vi "Change.vi"(6 "OldVal":variant, 8 "error in (no error)":errorcluster, 9 "NewVal":variant, 10 "Control Index":i32=-1, 11 "UndoObject in":refnum<class "UndoObject.lvclass">) -> (0 "error out":errorcluster, 1 "Redo Enable":bool, 2 "Undo Enable":bool, 3 "UndoObject out":refnum<class "UndoObject.lvclass">)   [LabVIEW 2015, in "UndoLibrary.lvlib" / "UndoObject.lvclass"]
doc: "This VI stores the changes produced in the controls. The maximum number of change is corresponding to the size of the buffer."
uses:
  UndoObject.lvclass
  UndoObject.lvclass/UndoObject.ctl
  Support VIs/DataClass/Controls/cluster_Control Value.ctl
  Support VIs/DataClass/DataObject.lvclass/DataObject.ctl
  <vilib>/Utility/error.llb/Error Cluster From Error Code.vi
  <vilib>/ErrorRing/Error Ring.xnode
  Support VIs/DataClass/DataObject.lvclass
  QueueOperations/QueueOperations.lvlib
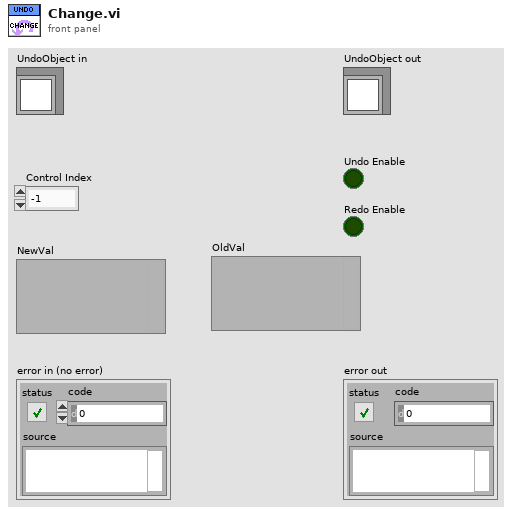
[diagram p1: front panel]
types:
  T1 = typedef "UndoLibrary.lvlib/DataObject.lvclass/cluster_Control Value.ctl" = cluster{"Index":i32, "Variant Data":variant}
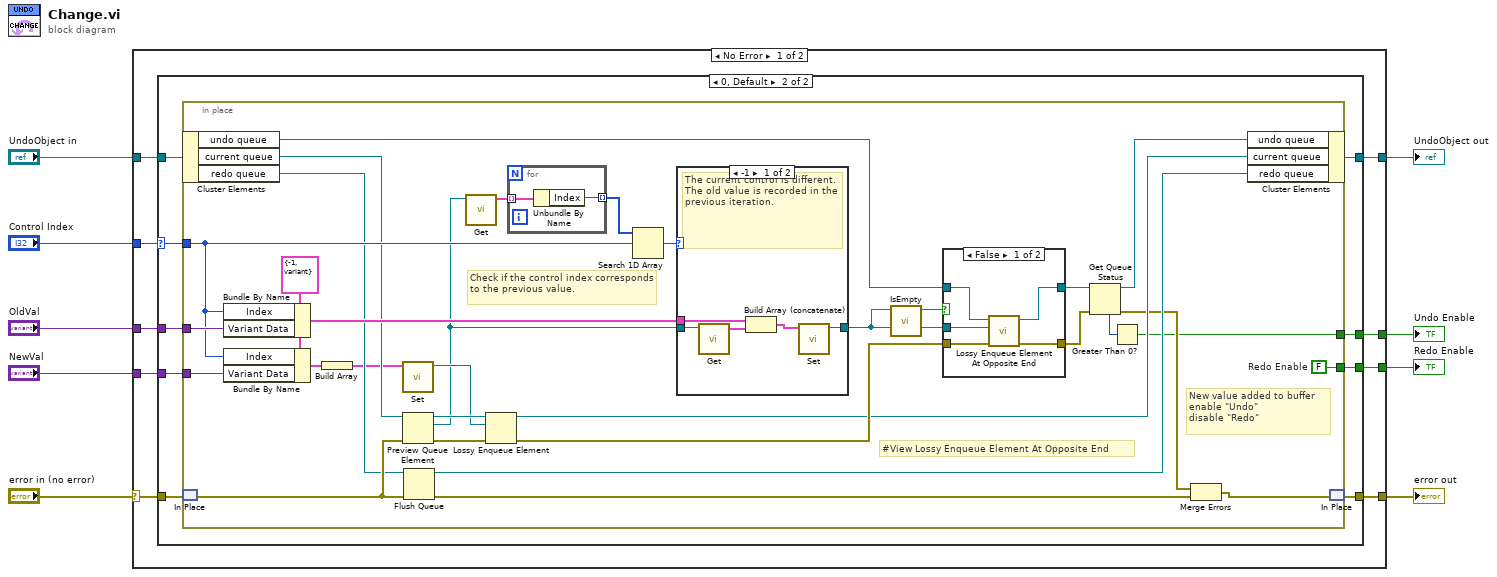
[diagram p0: block diagram]
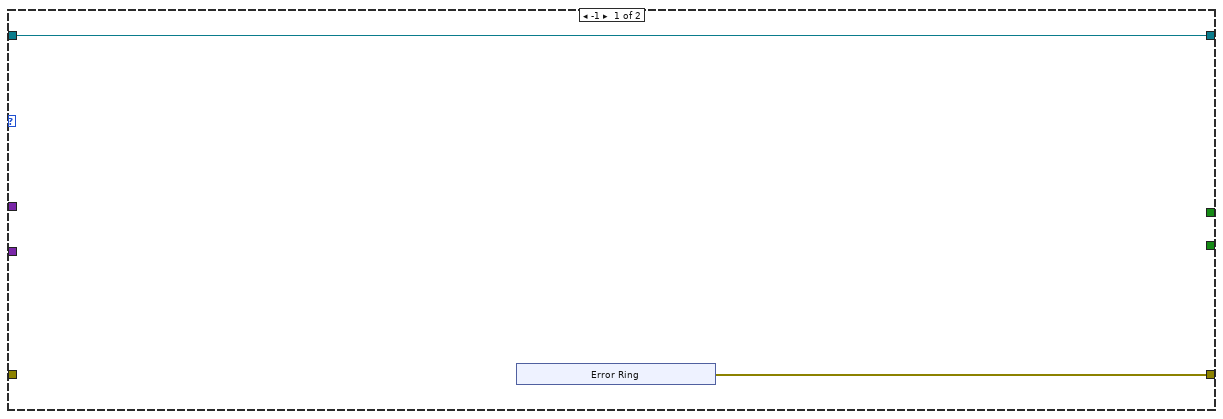
[diagram p2: hidden frame]
diagram:
  n1 = case shown="No Error" "error in (no error)" {
    selector: "error in (no error)" -> [w15 w82]
    tunnel: "OldVal" -> [w18 _]
    tunnel: "NewVal" -> [w17 _]
    tunnel: "Control Index" -> [w16 _]
    tunnel: "UndoObject in" -> [w13 w81]
    tunnel: [w12 w81] -> w1
    tunnel: [w14 w82] -> w5
    tunnel: [w11 _] -> w4
    tunnel: [w10 _] -> w3
    frame No Error {
      n2 = case shown="0, Default" w16 {
        selector: w16 -> [_ w31]
        tunnel: w18 -> [_ w33]
        tunnel: w17 -> [_ w32]
        tunnel: w15 -> [_ w30]
        tunnel: [w19 w29] -> w14
        tunnel: w13 -> [w20 w28]
        tunnel: [w20 w27] -> w12
        tunnel: [_ w26] -> w11
        tunnel: [_ w25] -> w10
        frame -1 {
          n3 = xnode "Error Ring"() -> ("error out"=w19:errorcluster)
        }
        frame 0, Default {
          n4 = in-place {
            in-place-border: w33 -> [w59]
            in-place-border: w32 -> [w58]
            in-place-border: w31 -> [w56]
            in-place-border: [w41] -> w26
            in-place-border: [w40] -> w25
            w40 = FALSE  # Redo Enable
            w63 = T1 {"Index"=-1, "Variant Data"=variant} ("Control Value")
            # "Check if the control index corresponds to the previous value."
            # "New value added to buffer\nenable \"Undo\"\ndisable \"Redo\""
            # "#View Lossy Enqueue Element At Opposite End"
            n5 = in-place-cluster #1(w28) -> ("undo queue"=w51:refnum<queue>, "current queue"=w50:refnum<queue>, "redo queue"=w49:refnum<queue>)
            n6 = in-place-match #2(w30) -> (w53:errorcluster)
            n7 = Bundle By Name(cluster=w63, "Index"=w56, "Variant Data"=w59) -> (w60:T1)
            n8 = Bundle By Name(cluster=w63, "Index"=w56, "Variant Data"=w58) -> (w57:T1)
            n9 = Build Array(w57) -> (w39:T1[])
            n10 = call "Set.vi"("Conrol Value[]"=w39) -> ("DataObject out"=w38:refnum<class "DataObject.lvclass">)  [unwired: 9 in, 1 out]
            n11 = Preview Queue Element(queue=w50, error in (no error)=w53) -> (queue out=w64:refnum<queue>, element=w37:refnum<class "DataObject.lvclass">, error out=w65:errorcluster)  [unwired: 1 in, 1 out]
            n12 = Flush Queue(queue=w49, error in (no error)=w53) -> (queue out=w44:refnum<queue>, error out=w55:errorcluster)  [unwired: 1 out]
            n13 = call "Get.vi"("DataObject in"=w37) -> ("Conrol Value[]"=w36:T1[])  [unwired: 9 in, 1 out]
            n14 = Lossy Enqueue Element(queue=w64, element=w38, error in (no error)=w65) -> (queue out=w48:refnum<queue>, error out=w54:errorcluster)  [unwired: 2 out]
            n15 = for {
              tunnel: [w67] -> w61 mode=indexing
              tunnel: w36 -> [w66] mode=indexing
              n16 = Unbundle By Name(w66) -> ("Index"=w67:i32)
            }
            n17 = Search 1D Array(1D array=w61, element=w56) -> (index of element=w62:i32)  [unwired: 1 in]
            n18 = case shown="-1" w62 {
              tunnel: w37 -> [w71 w73]
              tunnel: [w70 w73] -> w35
              tunnel: w60 -> [w72 _]
              frame -1 {
                # "The current control is different. The old value is recorded in the previous iteration."
                n19 = call "Get.vi"("DataObject in"=w71) -> ("Conrol Value[]"=w69:T1[])  [unwired: 9 in, 1 out]
                n20 = Build Array (concatenate)(w72, w69) -> (w68:T1[])
                n21 = call "Set.vi"("Conrol Value[]"=w68) -> ("DataObject out"=w70:refnum<class "DataObject.lvclass">)  [unwired: 9 in, 1 out]
              }
              frame 0, Default {
                # "It is the same control."
              }
            }
            n22 = call "IsEmpty.vi"("DataObject in"=w35) -> ("empty?"=w34:bool)  [unwired: 9 in, 1 out]
            n23 = case shown="False" w34 {
              tunnel: w51 -> [w78 w80]
              tunnel: [w75 w80] -> w47
              tunnel: w54 -> [w76 w79]
              tunnel: [w74 w79] -> w43
              tunnel: w35 -> [w77 _]
              frame False {
                n24 = call "Lossy Enqueue Element At Opposite End.vi"("error in (no error)"=w76, "element"=w77, "queue in"=w78) -> ("error out"=w74:errorcluster, "queue out"=w75:refnum<queue>)  [unwired: 5 in, 2 out]
              }
              frame True {
              }
            }
            n25 = Get Queue Status(queue=w47, error in (no error)=w43) -> (queue out=w46:refnum<queue>, error out=w42:errorcluster, # elements in queue=w45:i32)  [unwired: 1 in, 5 out]
            n26 = Greater Than 0?(x=w45) -> (x > 0?=w41:bool)
            n27 = Merge Errors(w42, w55) -> (w52:errorcluster)
            n28 = in-place-cluster #1("undo queue"=w46, "current queue"=w48, "redo queue"=w44) -> (w27:refnum<class "UndoObject.lvclass">)
            n29 = in-place-match #2(w52) -> (w29:errorcluster)
          }
        }
      }
    }
    frame Error {
    }
  }
  "error out" <- w5
  "Undo Enable" <- w4
  "Redo Enable" <- w3
  "UndoObject out" <- w1
